vi "init.vi"(0 "Digital Input Test in":refnum<class "Verify ILC Test.lvclass">, 1 "ReadILCStrategy":refnum<class "IReadILCStrategy.lvclass">, 2 "ConfigureILCStrategy":refnum<class "IConfigureILCStrategy.lvclass">, 3 "Expected":dbl, 4 "Tolerance":dbl, 5 "error in (no error)":errorcluster, 6 "Test Scenario":T1, 7 "Log":refnum<class "ITestLog.lvclass">, 8 "Signal Name":string) -> (14 "Digital Input Test out":refnum<class "Verify ILC Test.lvclass">, 19 "error out":errorcluster)   [LabVIEW 2015, in "Verify ILC Test.lvclass"]
uses:
  Verify ILC Test.lvclass
  Model/TestLog/ITestLog/ITestLog.lvclass
  Typedefs/TestScenarioTypes.ctl
  Model/ConfigureILCStrategy/IConfigureILCStrategy/IConfigureILCStrategy.lvclass
  Model/ReadILCStrategy/IReadILCStrategy/IReadILCStrategy.lvclass
  Verify ILC Test.lvclass/Verify ILC Test.ctl
  Typedefs/ILCBTTypedefs.lvlib
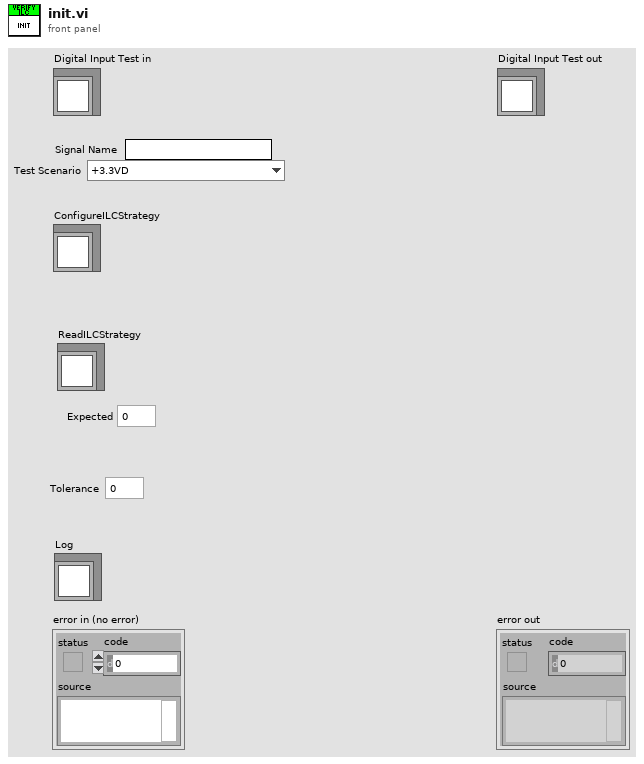
[diagram p1: front panel]
types:
  T1 = typedef "ILCBTTypedefs.lvlib/TestScenarioTypes.ctl" = enum16{"+3.3VD", "+5.1V", "+24V", "RELVALV1", "RELVALV2", "Verify DAC_A = -1.00A", "Verify DAC_A = -0.75A", "Verify DAC_A = -0.50A", "Verify DAC_A = -0.25A", "Verify DAC_A = 0.00A", "Verify DAC_A = 0.25A", "Verify DAC_A = 0.50A", "Verify DAC_A = 0.75A", "Verify DAC_A = 1.00A", "Verify DAC_B = -1.00A", "Verify DAC_B = -0.75A", "Verify DAC_B = -0.50A", "Verify DAC_B = -0.25A", "Verify DAC_B = 0.00A", "Verify DAC_B = 0.25A", "Verify DAC_B = 0.50A", "Verify DAC_B = 0.75A", "Verify DAC_B = 1.00A", "Set DAC_A = -1.00A", "Set DAC_A = -0.75A", "Set DAC_A = -0.50A", "Set DAC_A = -0.25A", "Set DAC_A = 0.00A", "Set DAC_A = 0.25A", "Set DAC_A = 0.50A", "Set DAC_A = 0.75A", "Set DAC_A = 1.00A", "Set DAC_B = -1.00A", "Set DAC_B = -0.75A", "Set DAC_B = -0.50A", "Set DAC_B = -0.25A", "Set DAC_B = 0.00A", "Set DAC_B = 0.25A", "Set DAC_B = 0.50A", "Set DAC_B = 0.75A", "Set DAC_B = 1.00A", "Set MTR_PWR = On", "Set MTR_PWR = Off", "Set OUTPUT = On", "Set OUTPUT = Off", "Verify OUTPUT = On", "Verify OUTPUT = Off", "Verify POWER = Ok", "Verify POWER = Fail", "Verify AMP1 = Ok", "Verify AMP1 = Fail", "Verify AMP2 = Ok", "Verify AMP2 = Fail"}
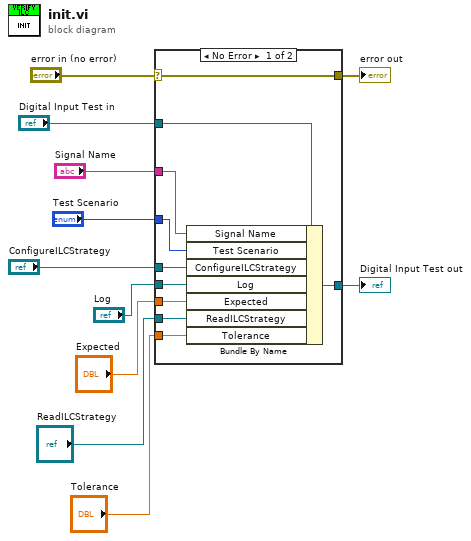
[diagram p0: block diagram]
diagram:
  n1 = case shown="No Error" "error in (no error)" {
    selector: "error in (no error)" -> [w21 w23]
    tunnel: [w21 w23] -> w10
    tunnel: [w17 w22] -> w8
    tunnel: "Digital Input Test in" -> [w20 w22]
    tunnel: "Signal Name" -> [w16 _]
    tunnel: "Test Scenario" -> [w15 _]
    tunnel: "ConfigureILCStrategy" -> [w18 _]
    tunnel: "Log" -> [w19 _]
    tunnel: "Expected" -> [w14 _]
    tunnel: "ReadILCStrategy" -> [w13 _]
    tunnel: "Tolerance" -> [w12 _]
    frame No Error {
      n2 = Bundle By Name(cluster=w20, "Signal Name"=w16, "Test Scenario"=w15, "ConfigureILCStrategy"=w18, "Log"=w19, "Expected"=w14, "ReadILCStrategy"=w13, "Tolerance"=w12) -> (w17:refnum<class "Verify ILC Test.lvclass">)
    }
    frame Error {
    }
  }
  "error out" <- w10
  "Digital Input Test out" <- w8
